vi "FlatToRichnixnet_grpc_WriteSignalXYRequest.vi"(5 "OutputClusterType":T1, 11 "InputCluster":T3) -> (3 "OutputCluster":T1)   [LabVIEW 2025, in "xnet-grpc_client.lvlib"]
uses:
  nixnet_grpc_WriteSignalXYRequest_Flat.ctl
  nidevice_grpc_Session_Flat.ctl
  nixnet_grpc_TimeOut.ctl
  nixnet_grpc_WriteSignalXYRequest.ctl
  nixnet_grpc_WriteSignalXYRequest_timeout_enum/nixnet_grpc_WriteSignalXYRequest_timeout_enum.lvclass
  nidevice_grpc_Session.ctl
  xnet-grpc_client.lvlib
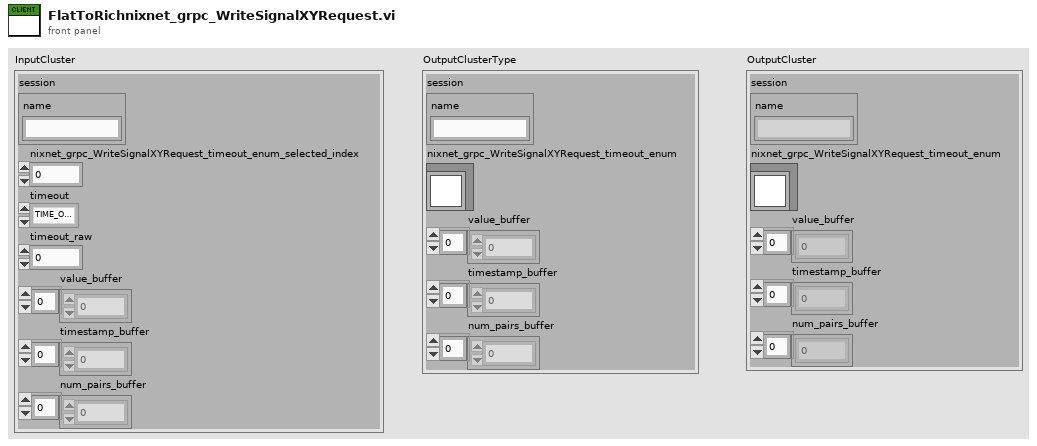
[diagram p1: front panel]
types:
  T1 = typedef "xnet-grpc_client.lvlib/nixnet_grpc_WriteSignalXYRequest.ctl" = cluster{"session":T2, "nixnet_grpc_WriteSignalXYRequest_timeout_enum":refnum<class "nixnet_grpc_WriteSignalXYRequest_timeout_enum.lvclass">, "value_buffer":dbl[], "timestamp_buffer":u64[], "num_pairs_buffer":u32[]}
  T2 = typedef "xnet-grpc_client.lvlib/nidevice_grpc_Session.ctl" = cluster{"name":string}
  T3 = typedef "xnet-grpc_client.lvlib/nixnet_grpc_WriteSignalXYRequest_Flat.ctl" = cluster{"session":T4, "nixnet_grpc_WriteSignalXYRequest_timeout_enum_selected_index":i32, "timeout":T5, "timeout_raw":dbl, "value_buffer":dbl[], "timestamp_buffer":u64[], "num_pairs_buffer":u32[]}
  T4 = typedef "xnet-grpc_client.lvlib/nidevice_grpc_Session_Flat.ctl" = cluster{"name":string}
  T5 = typedef "xnet-grpc_client.lvlib/nixnet_grpc_TimeOut.ctl" = enum32{"TIME_OUT_NONE", "TIME_OUT_INFINITE"}
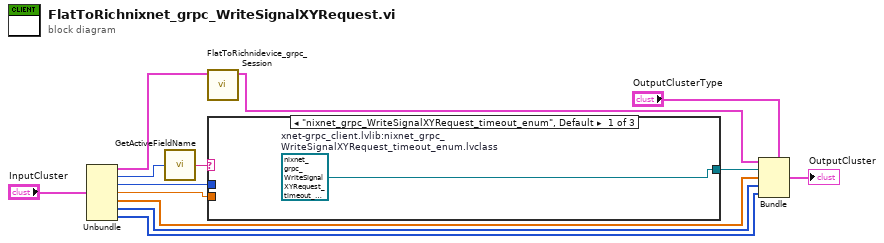
[diagram p0: block diagram]
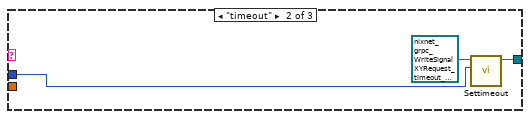
[diagram p2: hidden frame]
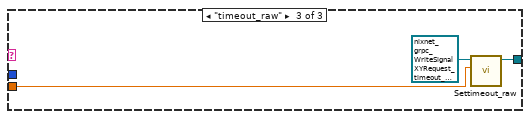
[diagram p3: hidden frame]
diagram:
  n1 = Unbundle "Unbundle"("InputCluster") -> ("session"=w10:T4, "nixnet_grpc_WriteSignalXYRequest_timeout_enum_selected_index"=w8:i32, "timeout"=w5:T5, "timeout_raw"=w4:dbl, "value_buffer"=w3:dbl[], "timestamp_buffer"=w2:u64[], "num_pairs_buffer"=w1:u32[])
  n2 = call "GetActiveFieldName.vi"("protobuf index"=w8) -> ("oneof field name"=w7:string)
  n3 = call "FlatToRichnidevice_grpc_Session.vi"("InputCluster"=w10) -> ("OutputCluster"=w9:T2)  [unwired: 10 in]
  n4 = case "nixnet_grpc_WriteSignalXYRequest_timeout_enum" shown="\"nixnet_grpc_WriteSignalXYRequest_timeout_enum\", Default" w7 {
    tunnel: [w14 w16 w19] -> w6
    tunnel: w5 -> [_ w17 _]
    tunnel: w4 -> [_ _ w20]
    frame "nixnet_grpc_WriteSignalXYRequest_timeout_enum", Default {
      w14 = refnum<class "nixnet_grpc_WriteSignalXYRequest_timeout_enum.lvclass"> refnum  # xnet-grpc_client.lvlib:nixnet_grpc_WriteSignalXYRequest_timeout_enum.lvclass
    }
    frame "timeout" {
      n5 = call "Settimeout.vi"("Set_Val"=w17, "OneOfTemplate in"=refnum<class "nixnet_grpc_WriteSignalXYRequest_timeout_enum.lvclass"> refnum) -> ("OneOfTemplate out"=w16:refnum<class "nixnet_grpc_WriteSignalXYRequest_timeout_enum.lvclass">)  [unwired: 8 in, 1 out]
    }
    frame "timeout_raw" {
      n6 = call "Settimeout_raw.vi"("Set_Val"=w20, "OneOfTemplate in"=refnum<class "nixnet_grpc_WriteSignalXYRequest_timeout_enum.lvclass"> refnum) -> ("OneOfTemplate out"=w19:refnum<class "nixnet_grpc_WriteSignalXYRequest_timeout_enum.lvclass">)  [unwired: 8 in, 1 out]
    }
  }
  n7 = Bundle "Bundle"(cluster="OutputClusterType", "session"=w9, "nixnet_grpc_WriteSignalXYRequest_timeout_enum"=w6, "value_buffer"=w3, "timestamp_buffer"=w2, "num_pairs_buffer"=w1) -> (→"OutputCluster":T1)
